vi "thermalResToCon.vi"(9 "Thermal Resistance":dbl, 10 "Area":dbl, 11 "Thickness":dbl) -> (3 "Thermal Conductivity":dbl)   [LabVIEW 2020]
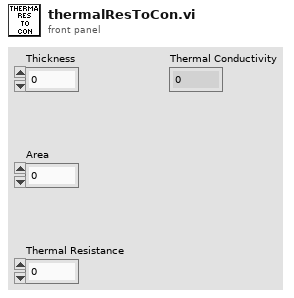
[diagram p1: front panel]
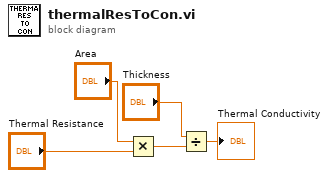
[diagram p0: block diagram]
diagram:
  n1 = Multiply(x="Area", y="Thermal Resistance") -> (x*y=w4:dbl)
  n2 = Divide(x="Thickness", y=w4) -> (x/y=→"Thermal Conductivity":dbl)
